vi "test Fails If Timestamps Are Not Equal (No Delta).vi"(8 "error in (no error)":errorcluster, 11 "TestCase in":refnum<class "Pass If Equal Timestamp Test Case.lvclass">) -> (0 "error out":errorcluster, 3 "TestCase out":refnum<class "Pass If Equal Timestamp Test Case.lvclass">)   [LabVIEW 2015, in "Pass If Equal Timestamp Test Case.lvclass"]
uses:
  Pass If Equal Timestamp Test Case.lvclass
  <vilib>/addons/_JKI Toolkits/VI Tester/TestCase.llb/TestCase.lvclass
  VITAC.lvlib
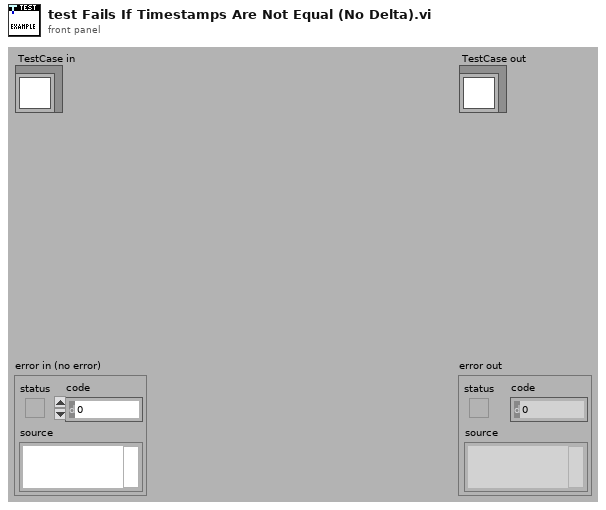
[diagram p1: front panel]
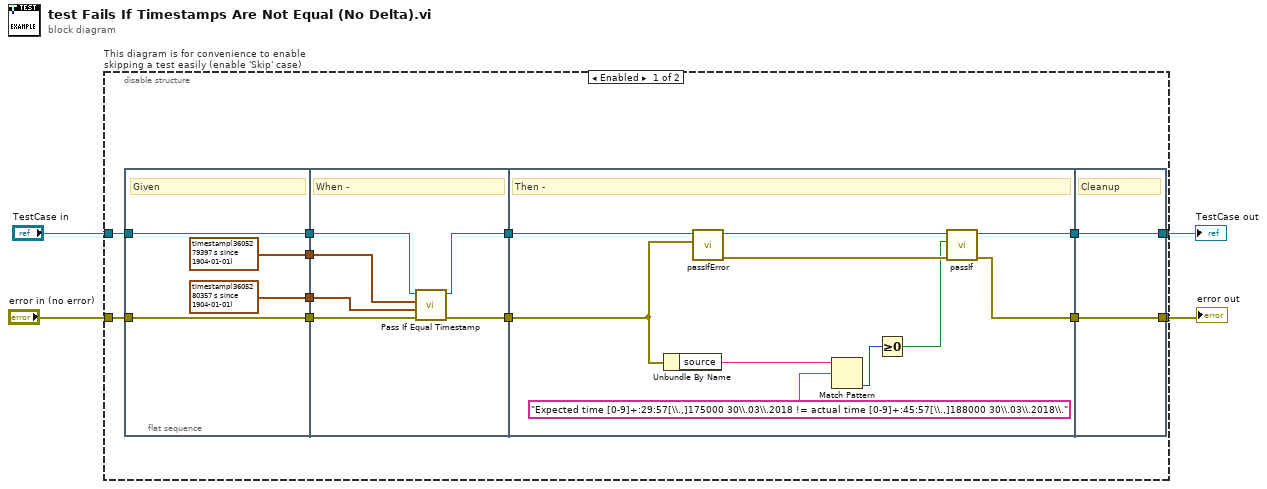
[diagram p0: block diagram]
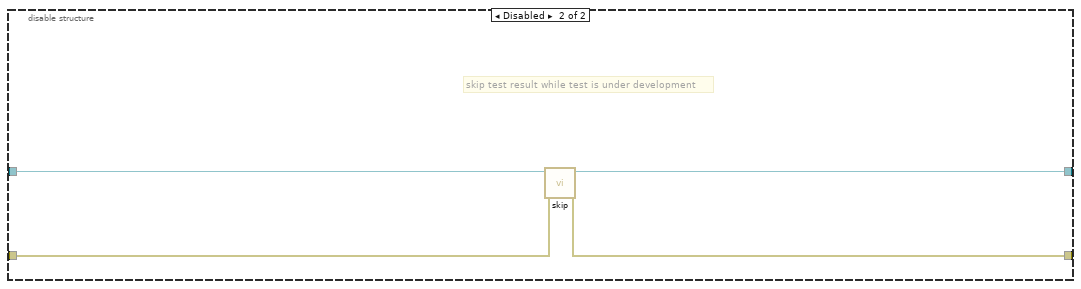
[diagram p2: hidden frame]
diagram:
  n1 = disable-structure "This diagram is for convenience to enable skipping a test easily (enable 'Skip' case)" shown="Enabled" {
    disable-tunnel: "TestCase in" -> [w7 w42]
    disable-tunnel: [w10 w40] -> w1
    disable-tunnel: [w9 w41] -> w3
    disable-tunnel: "error in (no error)" -> [w8 w39]
    frame Enabled {
      n2 = flat-sequence {
        tunnel: w8 -> [w19]
        tunnel: w7 -> [w20]
        tunnel: [w20] -> w16
        tunnel: [w19] -> w15
        tunnel: [timestamp(3605280357.188 s since 1904-01-01) ("Time Stamp")] -> w6
        tunnel: [timestamp(3605279397.175 s since 1904-01-01) ("Time Stamp")] -> w5
        tunnel: [w23] -> w14
        tunnel: [w25] -> w13
        tunnel: w16 -> [w24]
        tunnel: w15 -> [w26]
        tunnel: w6 -> [w21]
        tunnel: w5 -> [w22]
        tunnel: [w29] -> w12
        tunnel: w14 -> [w27]
        tunnel: w13 -> [w28]
        tunnel: [w30] -> w11
        tunnel: [w38] -> w9
        tunnel: w12 -> [w37]
        tunnel: w11 -> [w38]
        tunnel: [w37] -> w10
        frame #0 {
          # "Given"
        }
        frame #1 {
          # "When -"
          n3 = call "Pass If Equal Timestamp.vi"("error in (no error)"=w26, "actual timestamp"=w21, "expected timestamp"=w22, "TestCase in"=w24) -> ("error out"=w25:errorcluster, "TestCase out"=w23:refnum<class "Pass If Equal Timestamp Test Case.lvclass">)  [unwired: 6 in]
        }
        frame #2 {
          # "Then -"
          n4 = Unbundle By Name(w28) -> ("source"=w34:string)
          n5 = call-dynamic "passIfError.vi"("error"=w28, "TestCase in"=w27) -> ("error out"=w35:errorcluster, "TestCase out"=w36:refnum<class "Pass If Equal Timestamp Test Case.lvclass">)  [unwired: 8 in]
          n6 = Match Pattern(string=w34, regular expression="Expected time [0-9]+:29:57[\\.,]175000 30\\.03\\.2018 != actual time [0-9]+:45:57[\\.,]188000 30\\.03\\.2018\\.") -> (offset past match=w32:i32)  [unwired: 1 in, 3 out]
          n7 = Greater Or Equal To 0?(x=w32) -> (x >= 0?=w31:bool)
          n8 = call-dynamic "passIf.vi"("error in (no error)"=w35, "pass"=w31, "TestCase in"=w36) -> ("error out"=w30:errorcluster, "TestCase out"=w29:refnum<class "Pass If Equal Timestamp Test Case.lvclass">)  [unwired: 7 in]
        }
        frame #3 {
          # "Cleanup"
        }
      }
    }
    frame Disabled {
      # "skip test result while test is under development"
      n9 = call <vilib>:"skip.vi"("error in (no error)"=w39, "TestCase in"=w42) -> ("error out"=w41:errorcluster, "TestCase out"=w40:refnum<class "Pass If Equal Timestamp Test Case.lvclass">)  [unwired: 8 in]
    }
  }
  "error out" <- w3
  "TestCase out" <- w1
